vi "tsapp_configure_baudrate_lin.vi"(7 "AProtocol":i32, 8 "error in (no error)":errorcluster caption="错误输入（无错误）", 9 "ABaudrateKbps":sgl, 10 "AIdxChn":i32, 11 "路径输入":path) -> (0 "error out":errorcluster caption="错误输出", 2 "return":i32, 3 "路径输出":path)   [LabVIEW 2014]
doc: "Function Introduction :\nSet parameters such as baud rate for LIN channel\nCall location :\nBefore connecting hardware devices, set the parameters of the channel first\ninput parameter :\nAIdxChnq: Application Channel Number\nABaud rate Kbps: baud rate (kbps)\nAProtocol: baud rate (kbps)\nReturn value :\n==0: Connection successful\nOther: Check for error codes"
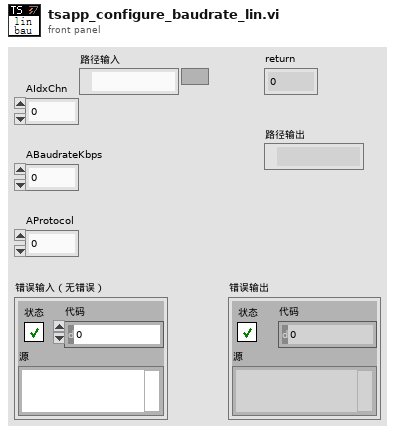
[diagram p1: front panel]
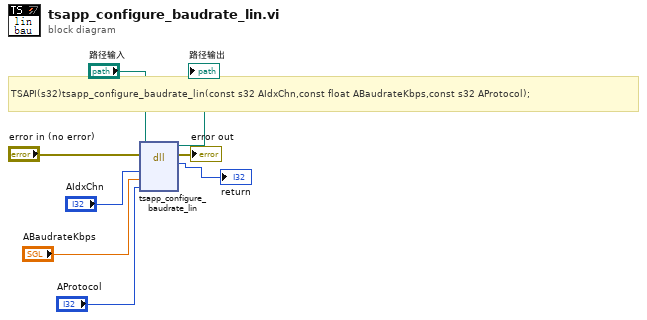
[diagram p0: block diagram]
diagram:
  # "TSAPI(s32)tsapp_configure_baudrate_lin(const s32 AIdxChn,const float ABaudrateKbps,const s32 AProtocol);"
  n1 = dll-call lib="D:/Work/LabVIEW Code/TSMaster Labview SDK/LabVIEW/LabVIEW-TSMasterAPI_CLN/TSMasterAPI_LabVIEW-2024-08-02 09-14-06/Not_organized_vi/TSMaster.*" fn="tsapp_configure_baudrate_lin"(path in="路径输入", error in="error in (no error)", "AIdxChn"="AIdxChn", "ABaudrateKbps"="ABaudrateKbps", "AProtocol"="AProtocol") -> (path out=→"路径输出":path, error out=→"error out":errorcluster, "返回类型"=→"return":i32)  [unwired: 4 in]
